vi "format SSN for display.vi"(5 "string":string) -> (2 "s? t:f":string)   [LabVIEW 2011]
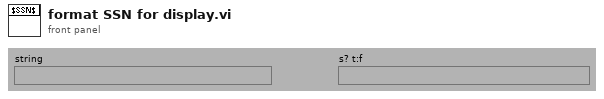
[diagram p1: front panel]
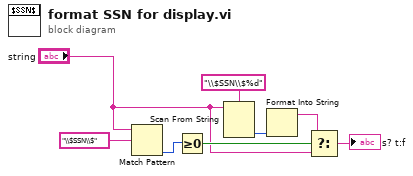
[diagram p0: block diagram]
diagram:
  n1 = Match Pattern(string="string", regular expression="\\$SSN\\$" ("format string")) -> (offset past match=w7:i32)  [unwired: 4 out]
  n2 = Greater Or Equal To 0?(x=w7) -> (x >= 0?=w6:bool)
  n3 = Scan From String(format string="\\$SSN\\$%d", input string="string") -> (output 1=w3:i32)  [unwired: 2 in, 4 out]
  n4 = Format Into String(w3) -> (resulting string=w2:string)  [unwired: 3 in, 1 out]
  n5 = Select(t=w2, s=w6, f="string") -> (s? t:f=→"s? t:f":string)
